vi "Destroy Client.vi"(8 "error in":errorcluster, 11 "gRPC ID":T1) -> (0 "error out":errorcluster)   [LabVIEW 2021, in "CoreGrpcClientWrapper.lvlib"]
uses:
  CoreGrpcClientWrapper.lvlib
  CIF_Plugin_Core_client/CIF_Plugin_Core_client.lvlib
  <vilib>/gRPC/LabVIEW gRPC Library/Shared/grpcId.ctl
  <vilib>/gRPC/LabVIEW gRPC Library/grpc-lvsupport-release.lvlib
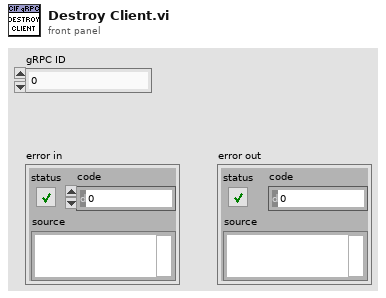
[diagram p1: front panel]
types:
  T1 = typedef "grpc-lvsupport-release.lvlib/grpcId.ctl" = u64
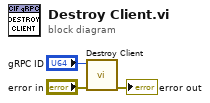
[diagram p0: block diagram]
diagram:
  n1 = call "Destroy Client.vi"("error in"="error in", "gRPC ID"="gRPC ID") -> ("error out"=→"error out":errorcluster)  [unwired: 9 in]
